vi "Rotation3D_Create_RotVector.vi"(11 "RotationVector":T1) -> (0 "Error":bool, 3 "Rotation3d":T2={"Q_quaternion"={"R"=1.0, "V"=[0.0, 0.0, 0.0]}})   [LabVIEW 2019, in "Trajectory_Library.lvlib"]
doc: "Constructs a Rotation3d from a rotation vector (3,1).\n\nInputs::\n -- rotationVector -- The rotation vector\n\nReturns:\n -- Rotation3d -- The created Rotation3d data cluster\n -- Error -- TRUE indicates an error occured."
uses:
  TypeDef/ROTATION3D.ctl
  TypeDef/QUATERNION.ctl
  <vilib>/Analysis/Matrix/Datatypes/RealMatrix.ctl
  Quaternion_Normalize.vi
  <vilib>/Analysis/_algsub.llb/Matrix Norm.vi
  <vilib>/Analysis/_algsub.llb/Real Matrix Norm.vi
  Quaternion_New_Default.vi
  <vilib>/Analysis/7linalg.llb/Create Special Matrix.vi
  <vilib>/Analysis/7linalg.llb/Create Special Real Matrix.vi
  Trajectory_Library.lvlib
  <vilib>/Analysis/Matrix/NI_Matrix.lvlib
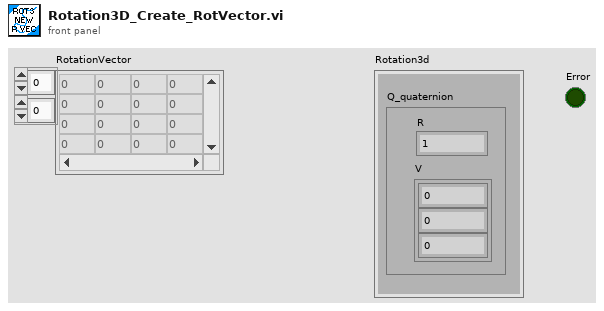
[diagram p1: front panel]
types:
  T1 = typedef "NI_Matrix.lvlib/RealMatrix.ctl" = dbl[][]
  T2 = typedef "Trajectory_Library.lvlib/ROTATION3D.ctl" = cluster{"Q_quaternion":T3}
  T3 = typedef "Trajectory_Library.lvlib/QUATERNION.ctl" = cluster{"R":dbl, "V":dbl[]}
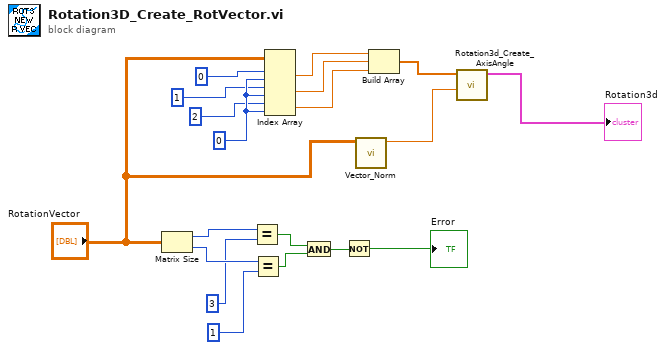
[diagram p0: block diagram]
diagram:
  w9 = 0 ("index (col)")
  n1 = Matrix Size(0:"RotationVector") -> (1:w19:i32, 2:w18:i32)
  n2 = Equal?(x=w19, y=3) -> (x = y?=w15:bool)
  n3 = Equal?(x=w18, y=1) -> (x = y?=w16:bool)
  n4 = Index Array(array="RotationVector", index (row) #1=0 ("index (row)"), index (col) #1=w9, index (row) #2=1 ("index (row)"), index (col) #2=w9, index (row) #3=2 ("index (row)"), index (col) #3=w9) -> (element #1=w6:dbl, element #2=w5:dbl, element #3=w4:dbl)
  n5 = And(x=w15, y=w16) -> (x .and. y?=w13:bool)
  n6 = Not(x=w13) -> (.not. x?=→"Error":bool)
  n7 = call "Vector_Norm.vi"("Input Vector"="RotationVector") -> ("norm"=w2:dbl)  [unwired: 10 in]
  n8 = Build Array(w6, w5, w4) -> (w11:dbl[])
  n9 = call "Rotation3d_Create_AxisAngle.vi"("Angle"=w2, "Axis Vector"=w11) -> ("Rotation3d"=→"Rotation3d":T2)  [unwired: 9 in]
